vi "Init_L16LinearActuator.vi"(3 "L16 Linear Actuator Port":refnum<visa-resource-name>="COM5") -> (0 "Connection":bool, 1 "L16 Linear Actuator":refnum<visa-resource-name>)   [LabVIEW 2022 SP3]
uses:
  <vilib>/Instr/_visa.llb/VISA Configure Serial Port (Instr).vi
panel:
  in  "error in (no error)":errorcluster
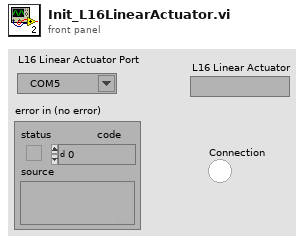
[diagram p1: front panel]
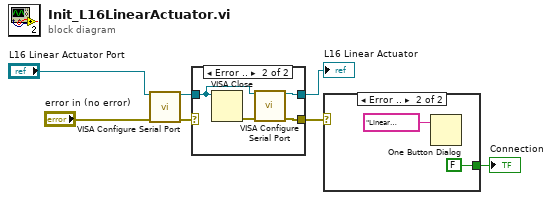
[diagram p0: block diagram]
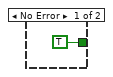
[diagram p2: hidden frame]
diagram:
  n1 = call-poly "VISA Configure Serial Port"("VISA resource name"="L16 Linear Actuator Port", "error in (no error)"="error in (no error)") -> ("VISA resource name out"=w6:refnum<visa-resource-name>, "error out"=w5:errorcluster)  [unwired: 12 in]
  n2 = case shown="Error .." w5 {
    selector: w5 -> [w9 _]
    tunnel: [w9 w12] -> w2
    tunnel: w6 -> [w8 w13]
    tunnel: [w8 w11] -> w3
    frame No Error {
    }
    frame Error {
      n3 = VISA Close(VISA resource name=w13) -> (error out=w10:errorcluster)  [unwired: 1 in]
      n4 = call-poly "VISA Configure Serial Port"("VISA resource name"=w13, "error in (no error)"=w10) -> ("VISA resource name out"=w11:refnum<visa-resource-name>, "error out"=w12:errorcluster)  [unwired: 12 in]
    }
  }
  "L16 Linear Actuator" <- w3
  n5 = case shown="Error .." w2 {
    tunnel: [TRUE FALSE] -> w1
    frame No Error {
    }
    frame Error {
      n6 = One Button Dialog(message="Linear Actuator connection error") -> ()  [unwired: 1 in, 1 out]
    }
  }
  "Connection" <- w1
